vi "fit angle data to line.vi"(7 "hrs":bool=TRUE, 10 "length":i32=2147483647, 11 "orbit fit":T1[](array[typedef])) -> (1 "degree/hr predicted":dbl, 2 "graphs (t, theta, theta_fit, dtheta_dt)":cluster{dbl[], dbl[]}[](array[cluster]), 3 "deg/hr":dbl, 5 "tmin":dbl)   [LabVIEW 2017]
uses:
  typedefs/orbit parameters with crossing info.ctl
  <vilib>/Analysis/baseanly.llb/Mean (DBL).vi
  <vilib>/Analysis/NI_AALBase.lvlib
  <vilib>/Analysis/NI_AALPro.lvlib
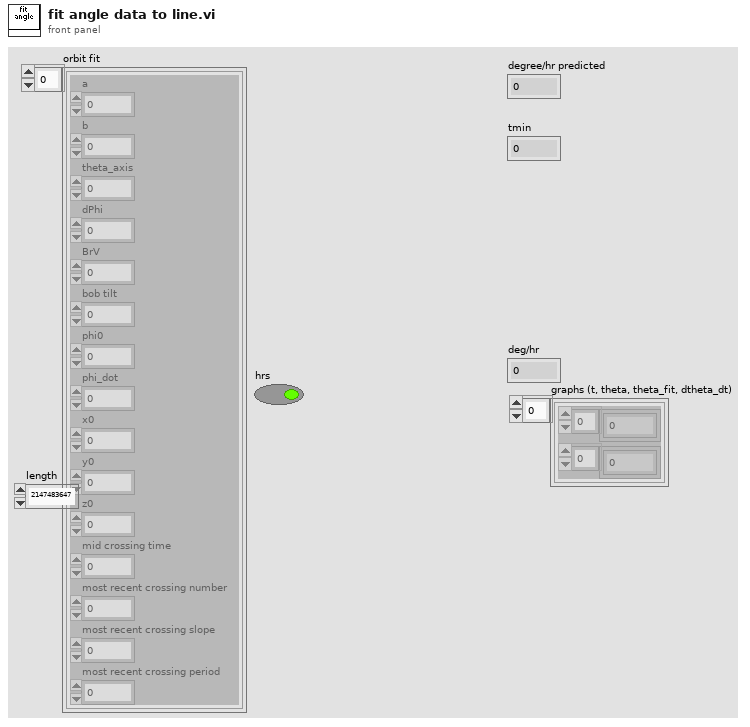
[diagram p1: front panel]
types:
  T1 = typedef "orbit parameters with crossing info.ctl" = cluster{"a":dbl, "b":dbl, "theta_axis":dbl, "dPhi":dbl, "BrV":dbl, "bob tilt":dbl, "phi0":dbl, "phi_dot":dbl, "x0":dbl, "y0":dbl, "z0":dbl, "mid crossing time":dbl, "most recent crossing number":dbl, "most recent crossing slope":dbl, "most recent crossing period":dbl}
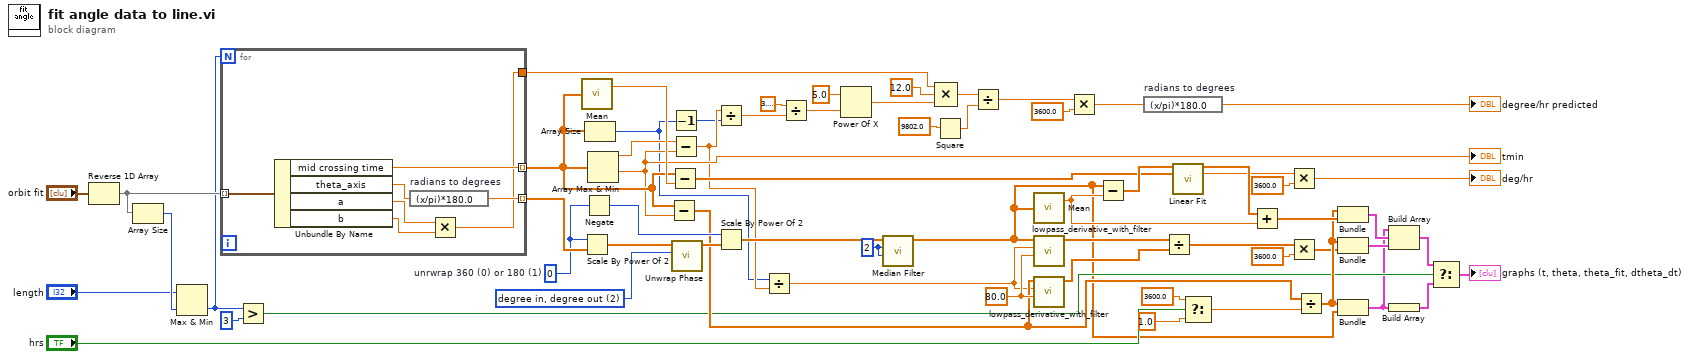
[diagram p0: block diagram]
diagram:
  w1 = 2 ("left rank")
  w38 = 80.0 ("sigma_time")
  w46 = i16 0  # unrwrap 360 (0) or 180 (1)
  w49 = 2 items=["radian in, radian out", "radian in, degree out", "degree in, degree out", "degree in, radian out"] ("phase unit")
  n1 = Reverse 1D Array(array="orbit fit") -> (reversed array=w63:T1[])
  n2 = Array Size(array=w63) -> (size(s)=w62:i32)
  n3 = Max & Min(x="length", y=w62) -> (min(x,y)=w9:i32)  [unwired: 1 out]
  n4 = for {
    N: w9 -> [_]
    tunnel: w63 -> [w71] mode=indexing
    tunnel: [w70] -> w40 mode=indexing
    tunnel: [w68] -> w50 mode=indexing
    tunnel: [w65] -> w27
    n5 = Unbundle By Name(w71) -> ("mid crossing time"=w70:dbl, "theta_axis"=w69:dbl, "a"=w67:dbl, "b"=w66:dbl)
    n6 = expression code="(x/pi)*180.0" "radians to degrees"(w69) -> (w68:dbl)
    n7 = Multiply(x=w67, y=w66) -> (x*y=w65:dbl)
  }
  n8 = Greater?(x=w9, y=3) -> (0:w7:bool)
  n9 = call-poly <vilib>:"Mean.vi"("X"=w40) -> ("mean"=w60:dbl)  [unwired: 1 out]
  n10 = Scale By Power Of 2(n=w46, x=w50) -> (x*2^n=w48:dbl[])
  n11 = Negate(x=w46) -> (-x=w45:i16)
  n12 = Array Size(array=w40) -> (size(s)=w13:i32)
  n13 = Array Max & Min(array=w40) -> (max value=w41:dbl, min value=w28:dbl)  [unwired: 2 out]
  "tmin" <- w28
  n14 = Subtract(x=w40, y=w28) -> (x-y=w32:dbl[])
  n15 = Subtract(x=w40, y=w60) -> (x-y=w53:dbl[])
  n16 = Decrement(x=w13) -> (x-1=w12:i32)
  n17 = Subtract(x=w41, y=w28) -> (x-y=w14:dbl)
  n18 = call <vilib>:"Unwrap Phase.vi"("phase unit"=w49, "Phase"=w48) -> ("Unwrapped Phase"=w47:dbl[])  [unwired: 8 in, 1 out]
  n19 = Divide(x=w14, y=w12) -> (x/y=w11:dbl)
  n20 = Scale By Power Of 2(n=w45, x=w47) -> (x*2^n=w39:dbl[])
  n21 = Divide(x=w13, y=w14) -> (x/y=w10:dbl)
  n22 = Divide(x=3.141592653589793, y=w11) -> (x/y=w20:dbl)
  n23 = Power Of X(1:w20, 2:5.0 ("y")) -> (0:w23:dbl)
  n24 = call <vilib>:"Median Filter.vi"("right rank"=w1, "left rank"=w1, "X"=w39) -> ("Filtered X"=w2:dbl[])  [unwired: 7 in, 1 out]
  n25 = Compound Arithmetic op=MULTIPLY(w27, 12.0 ("value"), w23) -> (w22:dbl)
  n26 = Square(x=9802.0) -> (x^2=w19:dbl)
  n27 = Divide(x=w22, y=w19) -> (x/y=w18:dbl)
  n28 = call-poly <vilib>:"Mean.vi"("X"=w2) -> ("mean"=w57:dbl)  [unwired: 1 out]
  n29 = call "lowpass_derivative_with_filter.vi"("sigma_time"=w38, "sampling frequency"=w10, "X"=w2) -> ("dX"=w36:dbl[])  [unwired: 8 in]
  n30 = call "lowpass_derivative_with_filter.vi"("sigma_time"=w38, "sampling frequency"=w10, "X"=w32) -> ("dX"=w35:dbl[])  [unwired: 8 in]
  n31 = Multiply(x=w18, y=3600.0) -> (x*y=w16:dbl)
  n32 = Subtract(x=w2, y=w57) -> (x-y=w59:dbl[])
  n33 = expression code="(x/pi)*180.0" "radians to degrees"(w16) -> (→"degree/hr predicted":dbl)
  n34 = Divide(x=w36, y=w35) -> (x/y=w34:dbl[])
  n35 = call <vilib>:"Linear Fit.vi"("Y"=w59, "X"=w53) -> ("Best Linear Fit"=w58:dbl[], "slope"=w56:dbl)  [unwired: 9 in, 3 out]
  n36 = Select(t=3600.0, s="hrs", f=1.0 ("t")) -> (s? t:f=w42:dbl)
  n37 = Add(x=w58, y=w57) -> (x+y=w52:dbl[])
  n38 = Multiply(x=w56, y=3600.0) -> (x*y=→"deg/hr":dbl)
  n39 = Multiply(x=w34, y=3600.0) -> (x*y=w31:dbl[])
  n40 = Divide(x=w32, y=w42) -> (x/y=w37:dbl[])
  n41 = Bundle(w37, w52) -> (w51:cluster{dbl[], dbl[]})  [unwired: 1 in]
  n42 = Bundle(w37, w31) -> (w33:cluster{dbl[], dbl[]})  [unwired: 1 in]
  n43 = Bundle(w37, "Filtered X"=w2) -> (w4:cluster{dbl[], "Filtered X":dbl[]})  [unwired: 1 in]
  n44 = Build Array(w4, w51, w33) -> (w6:cluster{dbl[], "Filtered X":dbl[]}[])
  n45 = Build Array(w4) -> (w3:cluster{dbl[], "Filtered X":dbl[]}[])
  n46 = Select(t=w6, s=w7, f=w3) -> (s? t:f=→"graphs (t, theta, theta_fit, dtheta_dt)":cluster{dbl[], "Filtered X":dbl[]}[])
